vi "Read Settings.vi"(7 "name":string, 8 "error in (no error)":errorcluster, 11 "refnum":T1) -> (0 "error out":errorcluster, 1 "value":T2, 2 "found?":bool, 3 "refnum out":T1)   [LabVIEW 2017, in "DSF Configuration API.lvlib"]
doc: "Reads a value associated with a key in a specified section from the configuration data identified by <B>refnum</B>. If the key does not exist, the VI returns the default value. This VI supports multibyte characters in strings. Wire data to the <B>default value</B> input to determine the polymorphic instance to use or manually select the instance."
uses:
  DSF Configuration API.lvlib
  Controls/DSF Settings Info.ctl
  Controls/DSF Config Data RefNum.ctl
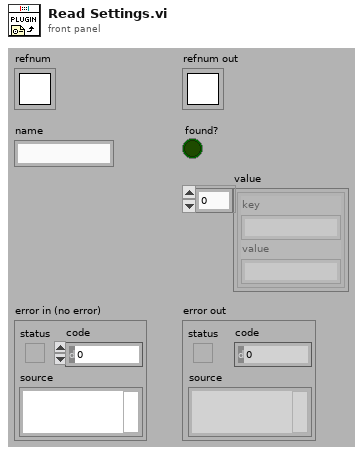
[diagram p1: front panel]
types:
  T1 = typedef "DSF Configuration API.lvlib/DSF Config Data RefNum.ctl" = refnum<k1>
  T2 = typedef "DSF Configuration API.lvlib/DSF Settings Info.ctl" = cluster{"key":string, "value":string}[]
  T3 = typedef "DSF Configuration API.lvlib/Config Queue.ctl" = refnum<queue>
  T4 = typedef "DSF Configuration API.lvlib/Config Data.ctl" = cluster{"dsf configuration":T5, "path":path, "dirty":bool}
  T5 = typedef "DSF Configuration API.lvlib/DSF Config.ctl" = cluster{"dsfversion":T6, "version":T6, "plugins":T7[], "groups":T10[], "transfers":T12[], "channels":T14[], "settings":T16[]}
  T6 = typedef "DSF Configuration API.lvlib/Version Info.ctl" = cluster{"major":u32, "minor":u32, "fix":u32, "build":string}
  T7 = typedef "DSF Configuration API.lvlib/DSF Plugin.ctl" = cluster{"id":string, "values":T8}
  T8 = typedef "DSF Configuration API.lvlib/DSF Plugin Info.ctl" = cluster{"type":string, "timing":T9, "group ids":string[], "settings id":string}
  T9 = typedef "DSF Configuration API.lvlib/DSF Timing Info.ctl" = cluster{"decimation":i32, "offset":i32}
  T10 = typedef "DSF Configuration API.lvlib/DSF Group.ctl" = cluster{"id":string, "values":T11}
  T11 = typedef "DSF Configuration API.lvlib/DSF Group Info.ctl" = cluster{"direction":i32, "timing":T9, "transfer ids":string[], "settings id":string}
  T12 = typedef "DSF Configuration API.lvlib/DSF Transfer.ctl" = cluster{"id":string, "values":T13}
  T13 = typedef "DSF Configuration API.lvlib/DSF Transfer Info.ctl" = cluster{"byte order":i32, "channel ids":string[], "settings id":string}
  T14 = typedef "DSF Configuration API.lvlib/DSF Channel.ctl" = cluster{"id":string, "values":T15}
  T15 = typedef "DSF Configuration API.lvlib/DSF Channel Info.ctl" = cluster{"count":i32, "offset":i32, "data type":i32, "resource path":string, "settings id":string}
  T16 = typedef "DSF Configuration API.lvlib/DSF Settings.ctl" = cluster{"id":string, "values":T2}
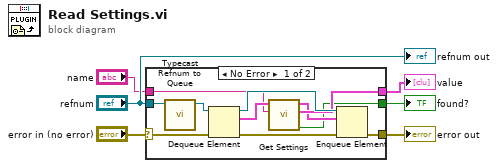
[diagram p0: block diagram]
diagram:
  n1 = case shown="No Error" "error in (no error)" {
    selector: "error in (no error)" -> [w17 w18]
    tunnel: "refnum" -> [w16 _]
    tunnel: [w12 w18] -> w4
    tunnel: "name" -> [w10 _]
    tunnel: [w9 _] -> w2
    tunnel: [w7 _] -> w1
    frame No Error {
      n2 = call "Typecast Refnum to Queue.vi"("refnum in"=w16) -> ("queue out"=w15:T3)  [unwired: 10 in]
      n3 = Dequeue Element(queue=w15, error in (no error)=w17) -> (queue out=w13:T3, element=w11:T4, error out=w14:errorcluster)  [unwired: 1 in, 1 out]
      n4 = call "Get Settings.vi"("id"=w10, "element"=w11) -> ("exists?"=w7:bool, "info"=w9:T2, "element out"=w8:T4)  [unwired: 6 in, 1 out]
      n5 = Enqueue Element(queue=w13, element=w8, error in (no error)=w14) -> (error out=w12:errorcluster)  [unwired: 1 in, 2 out]
    }
    frame Error {
    }
  }
  "error out" <- w4
  "found?" <- w1
  "value" <- w2
  "refnum out" <- "refnum"
